vi "engine.poststep.calc.vi"(7 "Procedure(pre)":variant[](array[variant])=[variant("procCLK"=variant(dbl 3802946268.2064614), "procIndex"=variant(dbl 2.0), "procIsRunning"=variant(bool TRUE), "procLabel"=variant(string "blink-2"), "procRegisterNumeric"=variant(dbl 3802946266.867457), "procReport"=variant(string "blink-2:3802946268,2>>2,_DELAY_COMPARE,1.3/2.0,STAY"), "procReportPast"=variant(string "blink-2:3802946268,2>>2,_DELAY_COMPARE,1.3/2.0,STAY")), variant("stepFunction"=variant(enum16{"__NO-OP", "_DELAY_LOAD", "_DELAY_COMPARE", "_COMPARE", "_JUMP", "_FINISH", "CLK_COMPARE", "PROC_START", "PROC_STOP", "PROC_ISRUN_COMPARE", "PROC_ISRUN_LOAD", "_IO_READ_IN", "_IO_WRITE_DOUT", "_IO_COMPARE", "Q_OPEN", "Q_WRITE", "Q_READ"} enum."_IO_WRITE_DOUT"), "stepIoPointer"=variant(string "dout2"), "stepIoState(str)"=variant(string "1:1"), "stepLabel"=variant(string "loop"), "stepPath"=variant(string "")), variant("stepFunction"=variant(enum16{"__NO-OP", "_DELAY_LOAD", "_DELAY_COMPARE", "_COMPARE", "_JUMP", "_FINISH", "CLK_COMPARE", "PROC_START", "PROC_STOP", "PROC_ISRUN_COMPARE", "PROC_ISRUN_LOAD", "_IO_READ_IN", "_IO_WRITE_DOUT", "_IO_COMPARE", "Q_OPEN", "Q_WRITE", "Q_READ"} enum."_DELAY_LOAD"), "stepLabel"=variant(string "")), variant("stepFunction"=variant(enum16{"__NO-OP", "_DELAY_LOAD", "_DELAY_COMPARE", "_COMPARE", "_JUMP", "_FINISH", "CLK_COMPARE", "PROC_START", "PROC_STOP", "PROC_ISRUN_COMPARE", "PROC_ISRUN_LOAD", "_IO_READ_IN", "_IO_WRITE_DOUT", "_IO_COMPARE", "Q_OPEN", "Q_WRITE", "Q_READ"} enum."_DELAY_COMPARE"), "stepSetpoint"=variant(cluster{"comparison":string, "Y":dbl} {"comparison"="", "Y"=2.0})), variant("stepFunction"=variant(enum16{"__NO-OP", "_DELAY_LOAD", "_DELAY_COMPARE", "_COMPARE", "_JUMP", "_FINISH", "CLK_COMPARE", "PROC_START", "PROC_STOP", "PROC_ISRUN_COMPARE", "PROC_ISRUN_LOAD", "_IO_READ_IN", "_IO_WRITE_DOUT", "_IO_COMPARE", "Q_OPEN", "Q_WRITE", "Q_READ"} enum."_JUMP"), "stepLabel"=variant(string ""), "stepPointer"=variant(string "loop"))], 8 "error in":errorcluster, 9 "isRunning?(T)":bool=TRUE, 10 "Next State in":cluster{"CMD":T1, "data":variant}={"CMD"=enum."JUMP", "data"=variant}, 11 "HeaderElement in":cluster{variant[]}) -> (0 "error out":errorcluster, 3 "Procedure Out":variant[](array[variant]))   [LabVIEW 2024]
uses:
  controls/typeCmdPostStepFunc.ctl
  controls/typeProcVarientName.ctl
  Polymorphics/variantCtrlNumber.vi
  Polymorphics/variantCtrlString.vi
  proc.util.validateParamExist.vi
  util.error.create.vi
  controls/typeStepVarients.ctl
panel:
  out "String Value":string
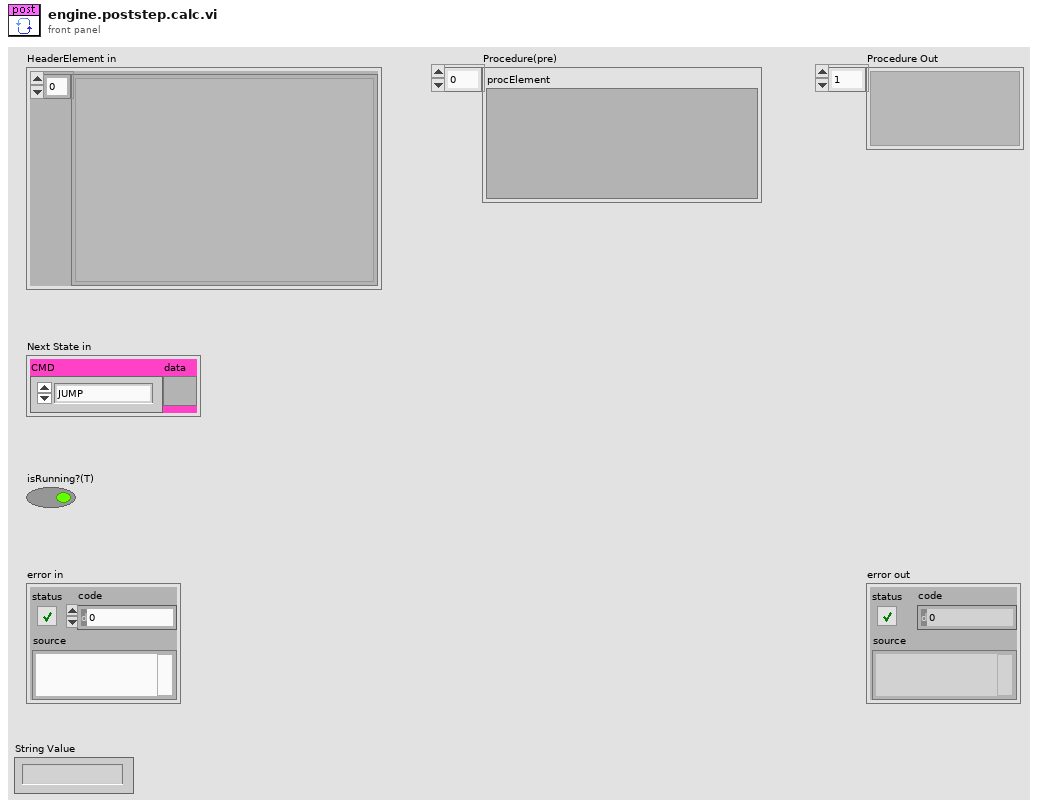
[diagram p1: front panel]
types:
  T1 = typedef "typeCmdPostStepFunc.ctl" = enum16{"NEXT", "PREV", "JUMP", "STAY", "COMPLETE", "ENGCALL.PROC.START", "ENGCALL.PROC.STOP", "ENGCALL.PROC.COMPLETION-CHECK", "ENGCALL.PROC.INIT", "ERROR"}
  T2 = typedef "typeProcVarientName.ctl" = enum16{"procNameID", "procModuleID", "procPath", "procIsRunning", "procIndex", "procModule", "procRegisterNumeric", "procRegisterString", "procReport", "procReportPrev", "procCLK", "procStepPointer", "procType"}
  T3 = typedef "typeStepVarients.ctl" = enum16{"stepNameID", "stepFunction", "stepReport", "stepSetpoint", "stepPointer", "stepProcPointer", "stepIoPointer", "stepIoValue", "stepFilePointer", "stepMessage", "stepTimeString", "stepNumReg", "stepStrReg", "stepSeconds", "stepUnitDoseParams", "stepUnitIndex"}
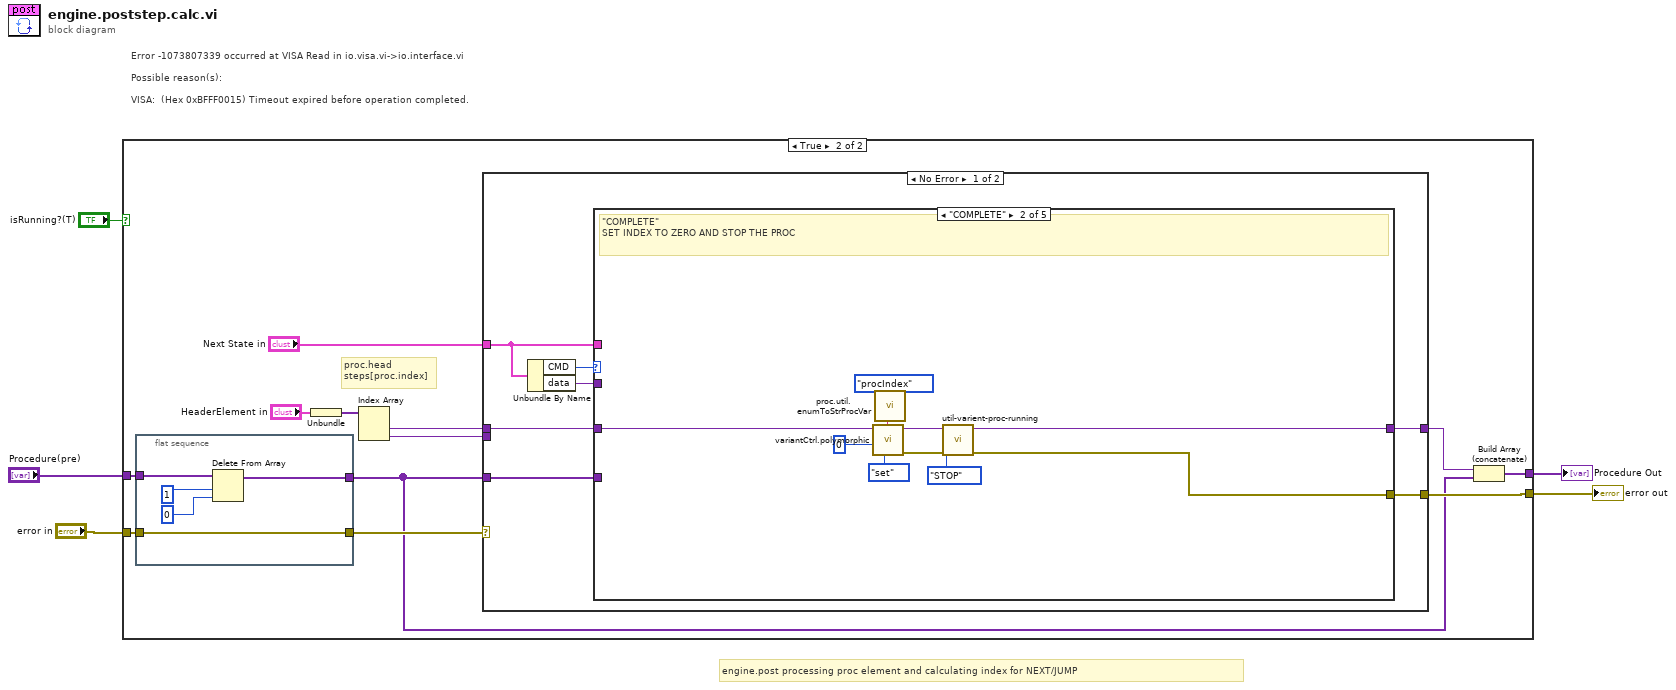
[diagram p0: block diagram]
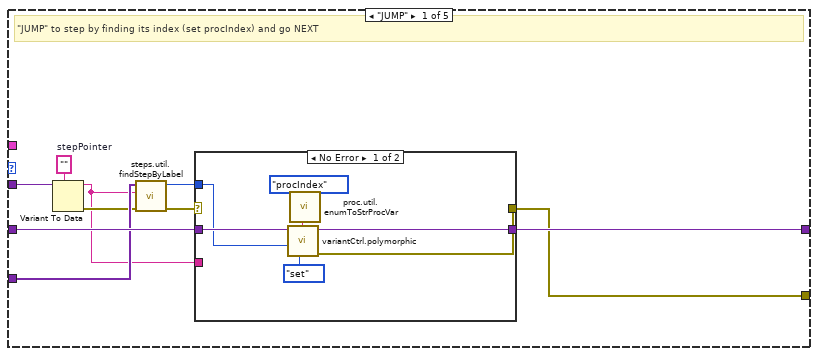
[diagram p3: hidden frame]
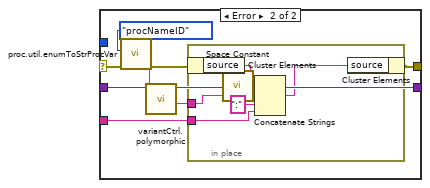
[diagram p4: hidden frame]
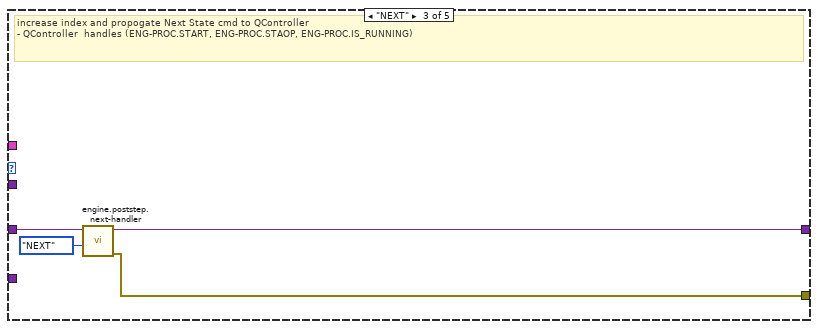
[diagram p5: hidden frame]
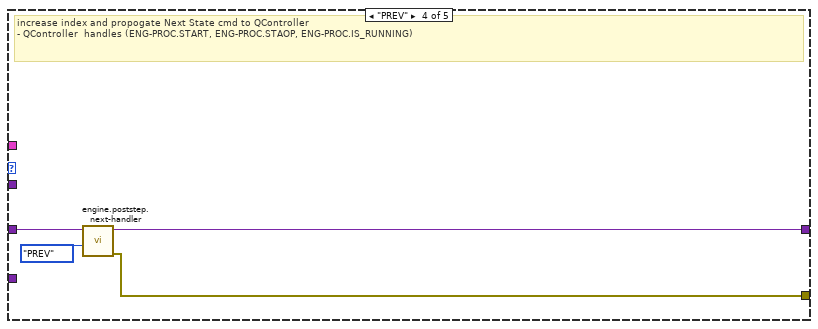
[diagram p6: hidden frame]
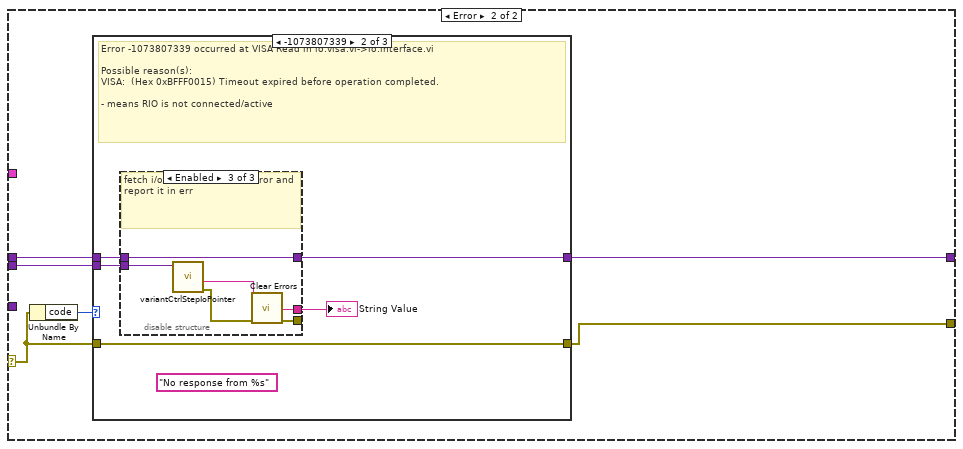
[diagram p8: hidden frame]
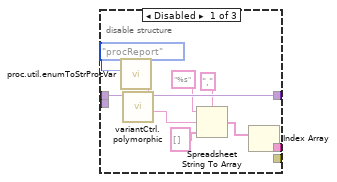
[diagram p10: hidden frame]
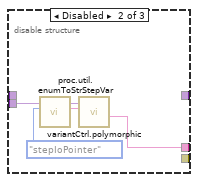
[diagram p11: hidden frame]
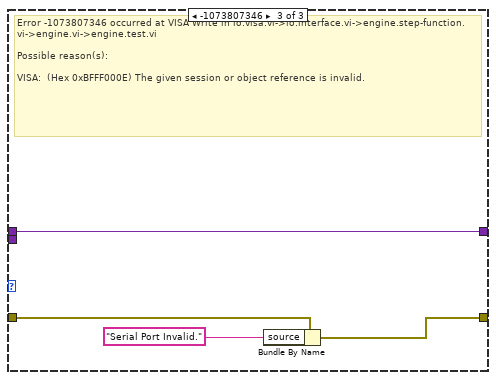
[diagram p12: hidden frame]
diagram:
  # "Error -1073807339 occurred at VISA Read in io.visa.vi->io.interface.vi\n\nPossible reason(s):\n\nVISA:  (Hex 0xBFFF0015) Timeout expired before operation completed."
  # "engine.post processing proc element and calculating index for NEXT/JUMP"
  n1 = case shown="True" "isRunning?(T)" {
    tunnel: [_ w18] -> w5
    tunnel: [w6 w11] -> w4
    tunnel: "Procedure(pre)" -> [w6 w8]
    tunnel: "error in" -> [_ w7]
    frame False {
    }
    frame True {
      # "proc.head \nsteps[proc.index]"
      n2 = flat-sequence {
        tunnel: [w112] -> w14
        tunnel: [w114] -> w9
        tunnel: w8 -> [w113]
        tunnel: w7 -> [w112]
        frame #0 {
          n3 = Delete From Array(array=w113, length=1, index=0) -> (array with subset deleted=w114:variant[])  [unwired: 1 out]
        }
      }
      n4 = Unbundle("HeaderElement in") -> (w16:variant[])
      n5 = Index Array(array=w16) -> (element #1=w13:variant, element #2=w10:variant)  [unwired: 2 in]
      n6 = case shown="No Error" w14 {
        selector: w14 -> [_ w79]
        tunnel: w13 -> [w25 w78]
        tunnel: "Next State in" -> [w20 _]
        tunnel: [w24 w80] -> w18
        tunnel: [w23 w77] -> w12
        tunnel: w10 -> [_ w76]
        tunnel: w9 -> [w19 _]
        frame No Error {
          n7 = Unbundle By Name(w20) -> ("CMD"=w22:T1, "data"=w21:variant)
          n8 = case shown="\"COMPLETE\"" w22 {
            tunnel: w25 -> [w35 w66 w69 w73 w75]
            tunnel: w19 -> [w34 _ _ _ _]
            tunnel: [w31 w58 w68 w72 _] -> w24
            tunnel: [w33 w59 w70 w74 w75] -> w23
            tunnel: w21 -> [w30 _ _ _ _]
            tunnel: w20 -> [_ _ _ _ _]
            frame "JUMP" {
              w29 = ""  # stepPointer
              # "\"JUMP\" to step by finding its index (set procIndex) and go NEXT"
              n9 = Variant To Data(type=w29, Variant=w30) -> (data=w26:string, error out=w28:errorcluster)  [unwired: 1 in]
              n10 = call "steps.util.findStepByLabel.vi"("error"=w28, "stepLabel"=w26, "steps in"=w34) -> ("error"=w27:errorcluster, "index"=w32:i32)  [unwired: 7 in]
              n11 = case shown="No Error" w27 {
                selector: w27 -> [_ w50]
                tunnel: w35 -> [w42 w49]
                tunnel: [w41 w47] -> w33
                tunnel: w32 -> [w40 _]
                tunnel: [w39 w48] -> w31
                tunnel: w26 -> [_ w43]
                frame No Error {
                  n12 = call "proc.util.enumToStrProcVar.vi"("Proc var"=typeProcVarientName."procIndex" ("name")) -> ("String"=w37:string)  [unwired: 10 in]
                  n13 = call-poly "variantCtrl.polymorphic.vi"("menu in (get)"=enum16{"get", "set"}."set", "number"=w40, "name in"=w37, "variant in"=w42) -> ("error out"=w39:errorcluster, "variant out"=w41:variant)  [unwired: 4 in, 2 out]
                }
                frame Error {
                  n14 = call "proc.util.enumToStrProcVar.vi"("Proc var"=typeProcVarientName."procNameID") -> ("String"=w46:string)  [unwired: 10 in]
                  n15 = call-poly "variantCtrl.polymorphic.vi"("name in"=w46, "Step in"=w49) -> ("String Value"=w44:string, "Step out"=w47:variant)  [unwired: 6 in, 2 out]
                  n16 = in-place {
                    in-place-border: w44 -> [w54]
                    in-place-border: w43 -> [w53]
                    n17 = in-place-cluster #1(w50) -> ("source"=w56:string)
                    n18 = call <vilib>:"Space Constant.vi"() -> ("String"=w55:string)
                    n19 = Concatenate Strings(w56, w55, w54, ":" ("string"), w53) -> (w51:string)
                    n20 = in-place-cluster #1("source"=w51) -> (w48:errorcluster)
                  }
                }
              }
            }
            frame "COMPLETE" {
              # "\"COMPLETE\"\nSET INDEX TO ZERO AND STOP THE PROC"
              n21 = call "proc.util.enumToStrProcVar.vi"("Proc var"=typeProcVarientName."procIndex" ("name")) -> ("String"=w64:string)  [unwired: 10 in]
              n22 = call-poly "variantCtrl.polymorphic.vi"("menu in (get)"=enum16{"get", "set"}."set", "number"=0 ("index"), "name in"=w64, "variant in"=w66) -> ("error out"=w61:errorcluster, "variant out"=w60:variant)  [unwired: 4 in, 2 out]
              n23 = call "util-varient-proc-running.vi"("error in"=w61, "Enum"=enum16{"START", "STOP"}."STOP", "Procedure in"=w60) -> ("error out"=w58:errorcluster, "Procedure out"=w59:variant)  [unwired: 7 in]
            }
            frame "NEXT" {
              # "increase index and propogate Next State cmd to QController\n- QController  handles (ENG-PROC.START, ENG-PROC.STAOP, ENG-PROC.IS_RUNNING)"
              n24 = call "engine.poststep.next-handler.vi"("NEXT/PREV"=enum16{"NEXT", "PREV"}."NEXT", "Proc Element in"=w69) -> ("error out"=w68:errorcluster, "Proc Element out"=w70:variant)  [unwired: 8 in]
            }
            frame "PREV" {
              # "increase index and propogate Next State cmd to QController\n- QController  handles (ENG-PROC.START, ENG-PROC.STAOP, ENG-PROC.IS_RUNNING)"
              n25 = call "engine.poststep.next-handler.vi"("NEXT/PREV"=enum16{"NEXT", "PREV"}."PREV", "Proc Element in"=w73) -> ("error out"=w72:errorcluster, "Proc Element out"=w74:variant)  [unwired: 8 in]
            }
            frame "STAY", Default {
              # "don't change the index go NEXT  index and propogate Next State cmd to QController\n- QController  handles (ENG-PROC.START, ENG-PROC.STAOP, ENG-PROC.IS_RUNNING)"
            }
          }
        }
        frame Error {
          n26 = Unbundle By Name(w79) -> ("code"=w81:i32)
          n27 = case shown="-1073807339" w81 {
            tunnel: [w83 w84 w109] -> w80
            tunnel: w79 -> [w83 w84 w111]
            tunnel: w78 -> [w82 w87 w108]
            tunnel: [w82 w88 w108] -> w77
            tunnel: w76 -> [_ w85 _]
            frame 0, Default {
            }
            frame -1073807339 {
              (unwired) "No response from %s" ("source")
              # "Error -1073807339 occurred at VISA Read in io.visa.vi->io.interface.vi\n\nPossible reason(s):\nVISA:  (Hex 0xBFFF0015) Timeout expired before operation completed.\n\n- means RIO is not connected/active"
              n28 = disable-structure shown="Enabled" {
                disable-tunnel: [w96 _ w104] -> w88
                disable-tunnel: w87 -> [w95 _ w104]
                disable-tunnel: [w89 w99 w106] -> w86
                disable-tunnel: w85 -> [_ w102 w107]
                disable-tunnel: [_ _ w103] -> _
                frame Disabled {
                  n29 = call "proc.util.enumToStrProcVar.vi"("Proc var"=typeProcVarientName."procReport" ("proc var")) -> ("String"=w97:string)  [unwired: 10 in]
                  n30 = call-poly "variantCtrl.polymorphic.vi"("name in"=w97, "Step in"=w95) -> ("String Value"=w92:string, "Step out"=w96:variant)  [unwired: 6 in, 2 out]
                  n31 = Spreadsheet String To Array(delimiter (Tab)=",", format string="%s", spreadsheet string=w92, array type (2D Dbl)=string[] []) -> (array=w90:string[])
                  n32 = Index Array(array=w90) -> (element=w89:string)  [unwired: 1 in]
                }
                frame Disabled {
                  n33 = call "proc.util.enumToStrStepVar.vi"("Step var"=typeStepVarients."stepIoPointer" ("proc var")) -> ("String"=w101:string)  [unwired: 10 in]
                  n34 = call-poly "variantCtrl.polymorphic.vi"("name in"=w101, "Step in"=w102) -> ("String Value"=w99:string)  [unwired: 6 in, 3 out]
                }
                frame Enabled {
                  # "fetch i/o label caused the error and report it in err"
                  n35 = call "variantCtrlStepIoPointer.vi"("StepElement in"=w107) -> ("error out"=w105:errorcluster, "I/O Pointer out"=w106:string)  [unwired: 7 in, 2 out]
                  n36 = call <vilib>:"Clear Errors.vi"("error in (no error)"=w105) -> ("error out"=w103:errorcluster)  [unwired: 5 in, 1 out]
                }
              }
              "String Value" <- w86
            }
            frame -1073807346 {
              # "Error -1073807346 occurred at VISA Write in io.visa.vi->io.interface.vi->engine.step-function.vi->engine.vi->engine.test.vi\n\nPossible reason(s):\n\nVISA:  (Hex 0xBFFF000E) The given session or object reference is invalid."
              n37 = Bundle By Name(cluster=w111, "source"="Serial Port Invalid.") -> (w109:errorcluster)
            }
          }
        }
      }
      n38 = Build Array (concatenate)(w12, w9) -> (w11:variant[])
    }
  }
  "Procedure Out" <- w4
  "error out" <- w5
